vi "Write Report Details.vi"(8 "error in (no error)":errorcluster, 10 "Report Details":T1, 11 "Report in":refnum<class "Report.lvclass">) -> (0 "error out":errorcluster, 3 "Report out":refnum<class "Report.lvclass">)   [LabVIEW 2019, in "Report.lvlib" / "Report.lvclass"]
uses:
  Report.lvclass
  Report.lvclass/Report.ctl
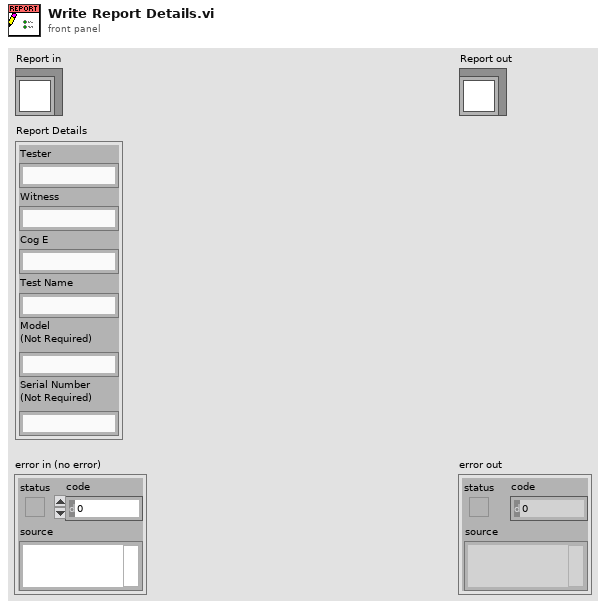
[diagram p1: front panel]
types:
  T1 = cluster{"Tester":string, "Witness":string, "Cog E":string, "Test Name":string, "Model\n(Not Required)":string, "Serial Number\n(Not Required)":string}
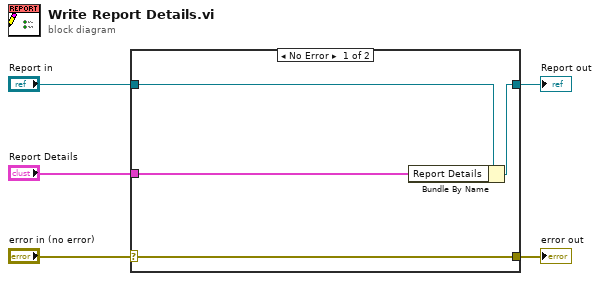
[diagram p0: block diagram]
diagram:
  n1 = case shown="No Error" "error in (no error)" {
    selector: "error in (no error)" -> [w9 w10]
    tunnel: [w9 w10] -> w4
    tunnel: [w7 w11] -> w2
    tunnel: "Report in" -> [w8 w11]
    tunnel: "Report Details" -> [w6 _]
    frame No Error {
      n2 = Bundle By Name(cluster=w8, "Report Details"=w6) -> (w7:refnum<class "Report.lvclass">)
    }
    frame Error {
    }
  }
  "error out" <- w4
  "Report out" <- w2
